vi "Stop Core.vi"(10 "final error code":i32, 11 "VHM-VNA_Hardware_Manager in":refnum<class "VHM-VNA_Hardware_Manager.lvclass">) -> (3 "VHM-VNA_Hardware_Manager out":refnum<class "VHM-VNA_Hardware_Manager.lvclass">)   [LabVIEW 2020, in "VHM-VNA_Hardware_Manager.lvlib" / "VHM-VNA_Hardware_Manager.lvclass"]
doc: "(<B>Filename</B>: Actor Framework.lvlib:Actor.lvclass:Stop Core.vi)\n\nDefines what the actor does before it stops. Use the <B>final error code</B> input to determine whether the actor shut down in response to an error.\n\nBy default, this method passes the Stop message along to all auto-stop nested actors. A descendant class may override this method to define additional behavior, such as shutting down any processes the actor initiated in its override of the Actor Core method."
uses:
  VHM-VNA_Hardware_Manager.lvclass
  <vilib>/ActorFramework/Actor/Actor.lvclass
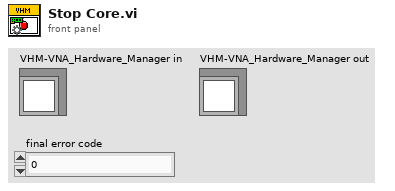
[diagram p1: front panel]
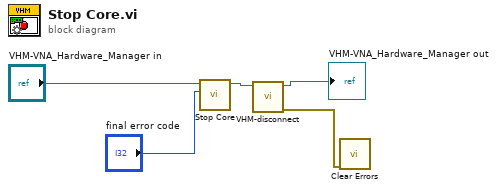
[diagram p0: block diagram]
diagram:
  n1 = call-parent "Stop Core.vi"("final error code"="final error code", "Actor in"="VHM-VNA_Hardware_Manager in") -> ("Actor out"=w3:refnum<class "VHM-VNA_Hardware_Manager.lvclass">)  [unwired: 9 in]
  n2 = call "VHM-disconnect.vi"("VHM-VNA_Hardware_Manager in"=w3) -> ("error out"=w1:errorcluster, "VHM-VNA_Hardware_Manager out"=→"VHM-VNA_Hardware_Manager out":refnum<class "VHM-VNA_Hardware_Manager.lvclass">)  [unwired: 9 in]
  n3 = call <vilib>:"Clear Errors.vi"("error in (no error)"=w1) -> ()  [unwired: 5 in, 2 out]
